vi "Transcriptor LabVIEW to VHDL code Step 1 and 2 Wires Declarations and Assignements.vi"(8 "error in":errorcluster, 11 "Diagram in":refnum<vi>) -> (1 "wires with enabled breakpoints":string[](array[string]), 2 "wires declarations":string[](array[string]), 3 "end loop refs.":string[](array[string]))   [LabVIEW 2018]
uses:
  <vilib>/Utility/miscctls.llb/LVBreakpointStatusEnum.ctl
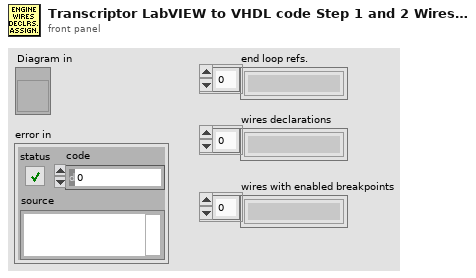
[diagram p1: front panel]
types:
  T1 = typedef "LVBreakpointStatusEnum.ctl" = enum8{"Cleared Break", "Enabled Break", "Disabled Break"}
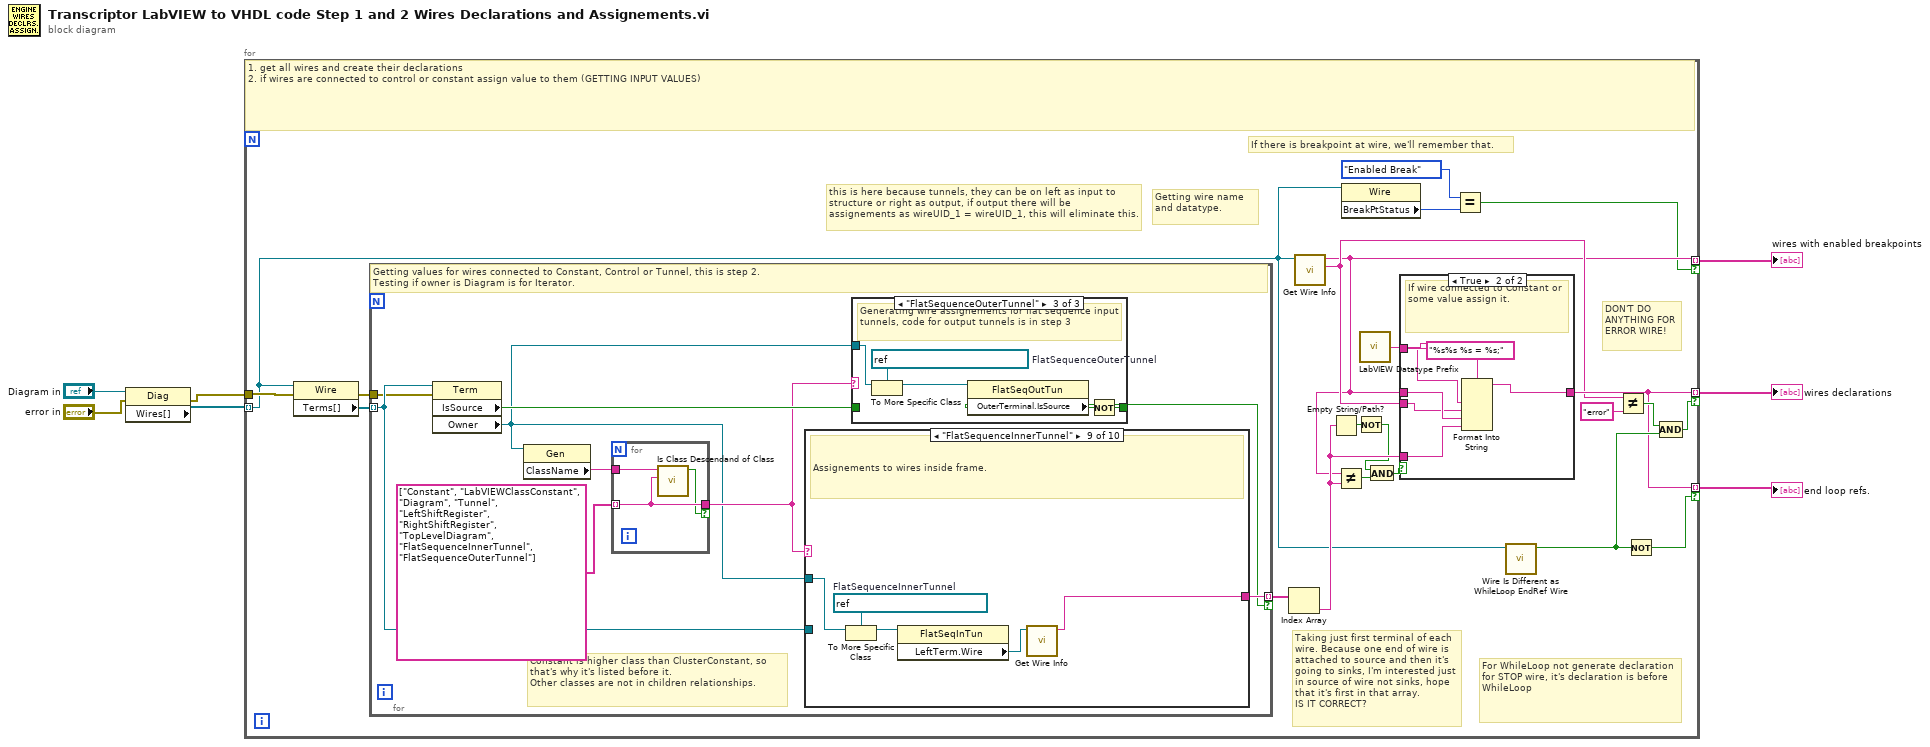
[diagram p0: block diagram]
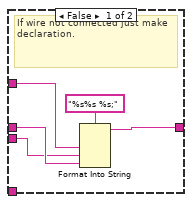
[diagram p2: hidden frame]
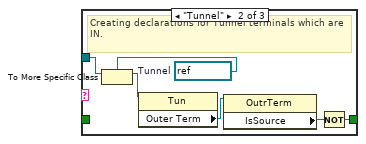
[diagram p4: hidden frame]
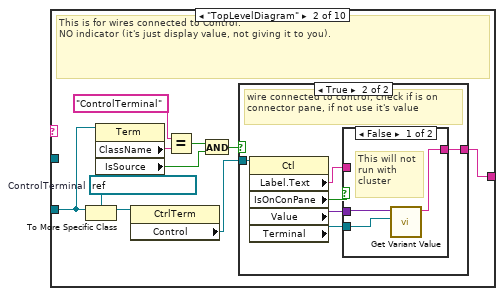
[diagram p6: hidden frame]
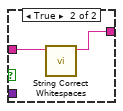
[diagram p8: hidden frame]
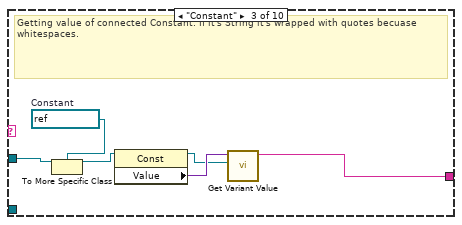
[diagram p9: hidden frame]
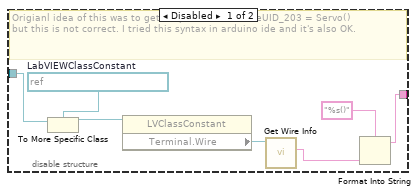
[diagram p11: hidden frame]
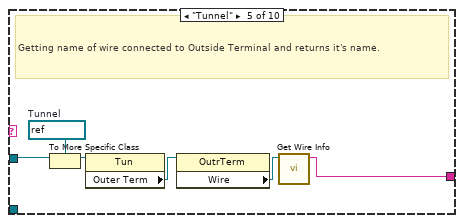
[diagram p12: hidden frame]
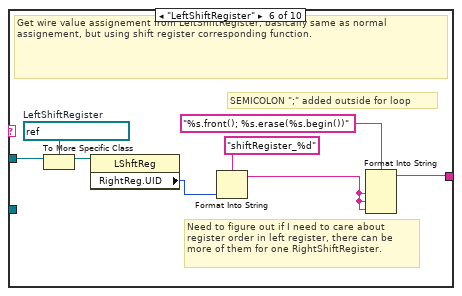
[diagram p13: hidden frame]
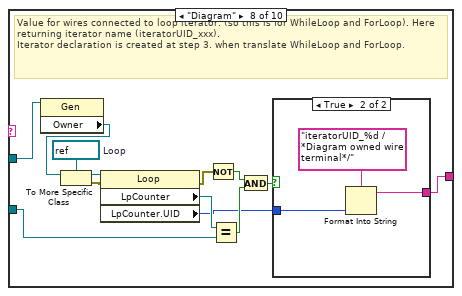
[diagram p15: hidden frame]
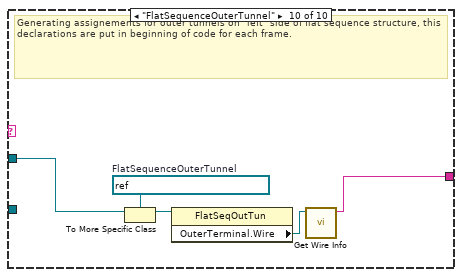
[diagram p17: hidden frame]
diagram:
  n1 = property class="Diag"(reference="Diagram in", error in="error in") -> (error out=w3:errorcluster, "Wires[]"=w2:refnum<vi>[])  [unwired: 1 out]
  n2 = for {
    tunnel: w2 -> [w12] mode=indexing
    tunnel: [w19] -> w7 mode=indexing if=w21
    tunnel: w3 -> [w25]
    tunnel: [w19] -> w6 mode=indexing if=w18
    tunnel: [w9] -> w1 mode=indexing if=w8
    # "If there is breakpoint at wire, we'll remember that."
    # "this is here because tunnels, they can be on left as input to structure or right as output, if output there will be assignements as wireUID_1 = wireUID_1, this will eliminate this."
    # "Getting wire name and datatype."
    # "For WhileLoop not generate declaration for STOP wire, it's declaration is before WhileLoop"
    # "Taking just first terminal of each wire. Because one end of wire is attached to source and then it's going to sinks, I'm interested just in source of wire not sinks, hope that it's first in that array.\nIS IT CORRECT?"
    # "DON'T DO ANYTHING FOR ERROR WIRE!"
    # "1. get all wires and create their declarations\n2. if wires are connected to control or constant assign value to them (GETTING INPUT VALUES)"
    n3 = property class="Wire"(reference=w12, error in=w25) -> (error out=w24:errorcluster, "Terms[]"=w29:refnum<vi>[])  [unwired: 1 out]
    n4 = for {
      tunnel: w29 -> [w48] mode=indexing
      tunnel: [w49] -> w28 mode=indexing if=w46
      tunnel: w24 -> [w47]
      # "Constant is higher class than ClusterConstant, so that's why it's listed before it.\nOther classes are not in children relationships."
      # "Getting values for wires connected to Constant, Control or Tunnel, this is step 2.\nTesting if owner is Diagram is for Iterator."
      n5 = property class="Term"(reference=w48, error in=w47) -> ("IsSource"=w45:bool, "Owner"=w41:refnum<vi>)  [unwired: 2 out]
      n6 = property class="Gen"(reference=w41) -> ("ClassName"=w43:string)  [unwired: 1 in, 2 out]
      n7 = for {
        tunnel: string[] ["Constant", "LabVIEWClassConstant", "Diagram", "Tunnel", "LeftShiftRegister", "RightShiftRegister", "TopLevelDiagram", "FlatSequenceInnerTunnel", "FlatSequenceOuterTunnel"] -> [w51] mode=indexing
        tunnel: w43 -> [w52]
        tunnel: [w51] -> w42 if=w50
        n8 = call "Is Class Descendand of Class.vi"("Parent ClassName"=w51, "ClassName"=w52) -> ("is Class descendant?"=w50:bool)  [unwired: 8 in, 1 out]
      }
      n9 = case shown="\"FlatSequenceInnerTunnel\"" w42 {
        tunnel: w41 -> [_ _ w91 w93 w105 w112 _ w127 w131 w136]
        tunnel: [_ w72 w88 w92 w101 w107 _ w117 w132 w138] -> w49
        tunnel: w48 -> [_ w70 _ _ _ _ _ w123 _ _]
        frame Default {
          # "If wire is not wired to anything from what I have to read value, output is default Variant value (hope that is empty Variant), and there will be just wire declaration without assignement in generated code."
        }
        frame "TopLevelDiagram" {
          w74 = refnum<vi> refnum  # ControlTerminal
          # "This is for wires connected to Control.\nNO indicator (it's just display value, not giving it to you)."
          n10 = To More Specific Class(target class=w74, reference=w70) -> (specific class reference=w73:refnum<vi>)  [unwired: 1 in, 1 out]
          n11 = property class="Term"(reference=w70) -> ("ClassName"=w69:string, "IsSource"=w65:bool)  [unwired: 1 in, 2 out]
          n12 = property class="CtrlTerm"(reference=w73) -> ("Control"=w68:refnum<vi>)  [unwired: 1 in, 2 out]
          n13 = Equal?(x="ControlTerminal", y=w69) -> (x = y?=w66:bool)
          n14 = And(x=w66, y=w65) -> (x .and. y?=w67:bool)
          n15 = case shown="True" w67 {
            tunnel: [_ w78] -> w72
            tunnel: w68 -> [_ w80]
            frame False {
              # "wire connected to indicator, do nothing"
            }
            frame True {
              # "wire connected to control, check if is on connector pane, if not use it's value"
              n16 = property class="Ctl"(reference=w80) -> ("Label.Text"=w79:string, "IsOnConPane"=w77:bool, "Value"=w76:variant, "Terminal"=w75:refnum<vi>)  [unwired: 1 in, 2 out]
              n17 = case shown="False" w77 {
                tunnel: w79 -> [_ w85]
                tunnel: [w82 w84] -> w78
                tunnel: w76 -> [w83 _]
                tunnel: w75 -> [w81 _]
                frame False {
                  # "This will not\nrun with\ncluster"
                  n18 = call "Get Variant Value.vi"("GObj Refnum"=w81, "Variant in"=w83) -> ("Variant value as string"=w82:string)  [unwired: 9 in]
                }
                frame True {
                  n19 = call "String Correct Whitespaces.vi"("String in"=w85) -> ("String out"=w84:string)  [unwired: 10 in]
                }
              }
            }
          }
        }
        frame "Constant" {
          w90 = refnum<vi> refnum  # Constant
          # "Getting value of connected Constant. If it's String it's wrapped with quotes becuase whitespaces."
          n20 = To More Specific Class(target class=w90, reference=w91) -> (specific class reference=w89:refnum<vi>)  [unwired: 1 in, 1 out]
          n21 = property class="Const"(reference=w89) -> (reference out=w86:refnum<vi>, "Value"=w87:variant)  [unwired: 1 in, 1 out]
          n22 = call "Get Variant Value.vi"("GObj Refnum"=w86, "Variant in"=w87) -> ("Variant value as string"=w88:string)  [unwired: 9 in]
        }
        frame "LabVIEWClassConstant" {
          # "For class constant connected to wire there is nothing to get, we have to in the end obtain just normal C++ object declaration ie. for Servo class:\nServo wireUID_203;"
          n23 = disable-structure shown="Enabled" {
            disable-tunnel: w93 -> [w100 _]
            disable-tunnel: [w95 _] -> w92
            frame Disabled {
              w99 = refnum<vi> refnum  # LabVIEWClassConstant
              # "Origianl idea of this was to get output as Servo wireUID_203 = Servo()\nbut this is not correct. I tried this syntax in arduino ide and it's also OK."
              n24 = To More Specific Class(target class=w99, reference=w100) -> (specific class reference=w98:refnum<vi>)  [unwired: 1 in, 1 out]
              n25 = property class="LVClassConstant"(reference=w98) -> ("Terminal.Wire"=w97:refnum<vi>)  [unwired: 1 in, 2 out]
              n26 = call "Get Wire Info.vi"("Wire"=w97) -> ("wire datatype"=w94:string)  [unwired: 9 in, 1 out]
              n27 = Format Into String(format string="%s()", w94) -> (resulting string=w95:string)  [unwired: 2 in, 1 out]
            }
            frame Enabled {
              # "Nothing to return, so in the end object wire declaration is without initilization (we are working normal memory of MCU NOT in stack!)"
            }
          }
        }
        frame "Tunnel" {
          w106 = refnum<vi> refnum  # Tunnel
          # "Getting name of wire connected to Outside Terminal and returns it's name."
          n28 = To More Specific Class(target class=w106, reference=w105) -> (specific class reference=w104:refnum<vi>)  [unwired: 1 in, 1 out]
          n29 = property class="Tun"(reference=w104) -> ("Outer Term"=w103:refnum<vi>)  [unwired: 1 in, 2 out]
          n30 = property class="OutrTerm"(reference=w103) -> ("Wire"=w102:refnum<vi>)  [unwired: 1 in, 2 out]
          n31 = call "Get Wire Info.vi"("Wire"=w102) -> ("wire label"=w101:string)  [unwired: 9 in, 1 out]
        }
        frame "LeftShiftRegister" {
          w114 = refnum<vi> refnum  # LeftShiftRegister
          # "SEMICOLON \";\" added outside for loop"
          # "Need to figure out if I need to care about register order in left register, there can be more of them for one RightShiftRegister."
          # "Get wire value assignement from LeftShiftRegister, basically same as normal assignement, but using shift register corresponding function."
          n32 = To More Specific Class(target class=w114, reference=w112) -> (specific class reference=w113:refnum<vi>)  [unwired: 1 in, 1 out]
          n33 = property class="LShftReg"(reference=w113) -> ("RightReg.UID"=w110:i32)  [unwired: 1 in, 2 out]
          n34 = Format Into String(format string="shiftRegister_%d", w110) -> (resulting string=w108:string)  [unwired: 2 in, 1 out]
          n35 = Format Into String(format string="%s.front(); %s.erase(%s.begin())", w108, w108, w108) -> (resulting string=w107:string)  [unwired: 2 in, 1 out]
        }
        frame "RightShiftRegister" {
          # "For RightShiftRegister there is nothing to do, no init value, so this left blank."
        }
        frame "Diagram" {
          w126 = refnum<vi> refnum  # Loop
          # "Value for wires connected to loop iterator. (so this is for WhileLoop and ForLoop). Here returning iterator name (iteratorUID_xxx).\nIterator declaration is created at step 3. when translate WhileLoop and ForLoop."
          n36 = property class="Gen"(reference=w127) -> ("Owner"=w115:refnum<vi>)  [unwired: 1 in, 2 out]
          n37 = To More Specific Class(target class=w126, reference=w115) -> (specific class reference=w125:refnum<vi>, error out=w122:errorcluster)  [unwired: 1 in]
          n38 = property class="Loop"(reference=w125, error in=w122) -> (error out=w121:errorcluster, "LpCounter"=w124:refnum<vi>, "LpCounter.UID"=w116:i32)  [unwired: 1 out]
          n39 = Not(x=w121) -> (.not. x?=w120:bool)
          n40 = Equal?(x=w124, y=w123) -> (x = y?=w119:bool)
          n41 = And(x=w120, y=w119) -> (x .and. y?=w118:bool)
          n42 = case shown="True" w118 {
            tunnel: [_ w130] -> w117
            tunnel: w116 -> [_ w128]
            frame False {
            }
            frame True {
              n43 = Format Into String(format string="iteratorUID_%d /*Diagram owned wire terminal*/", w128) -> (resulting string=w130:string)  [unwired: 2 in, 1 out]
            }
          }
        }
        frame "FlatSequenceInnerTunnel" {
          w135 = refnum<vi> refnum  # FlatSequenceInnerTunnel
          # "Assignements to wires inside frame."
          n44 = To More Specific Class(target class=w135, reference=w131) -> (specific class reference=w134:refnum<vi>)  [unwired: 1 in, 1 out]
          n45 = property class="FlatSeqInTun"(reference=w134) -> ("LeftTerm.Wire"=w133:refnum<vi>)  [unwired: 1 in, 2 out]
          n46 = call "Get Wire Info.vi"("Wire"=w133) -> ("wire label"=w132:string)  [unwired: 9 in, 1 out]
        }
        frame "FlatSequenceOuterTunnel" {
          w140 = refnum<vi> refnum  # FlatSequenceOuterTunnel
          # "Generating assignements for outer tunnels on \"left\" side of flat sequence structure, this declarations are put in beginning of code for each frame."
          n47 = To More Specific Class(target class=w140, reference=w136) -> (specific class reference=w139:refnum<vi>)  [unwired: 1 in, 1 out]
          n48 = property class="FlatSeqOutTun"(reference=w139) -> ("OuterTerminal.Wire"=w137:refnum<vi>)  [unwired: 1 in, 2 out]
          n49 = call "Get Wire Info.vi"("Wire"=w137) -> ("wire label"=w138:string)  [unwired: 9 in, 1 out]
        }
      }
      n50 = case shown="\"FlatSequenceOuterTunnel\"" w42 {
        tunnel: [w53 w54 w61] -> w46
        tunnel: w45 -> [w53 _ _]
        tunnel: w41 -> [_ w56 w62]
        frame Default {
          # "For all others Terminal.Owner don't need to do anything else."
        }
        frame "Tunnel" {
          w58 = refnum<vi> refnum  # Tunnel
          # "Creating declarations for Tunnel terminals which are IN."
          n51 = To More Specific Class(target class=w58, reference=w56) -> (specific class reference=w59:refnum<vi>)  [unwired: 1 in, 1 out]
          n52 = property class="Tun"(reference=w59) -> ("Outer Term"=w57:refnum<vi>)  [unwired: 1 in, 2 out]
          n53 = property class="OutrTerm"(reference=w57) -> ("IsSource"=w55:bool)  [unwired: 1 in, 2 out]
          n54 = Not(x=w55) -> (.not. x?=w54:bool)
        }
        frame "FlatSequenceOuterTunnel" {
          w63 = refnum<vi> refnum  # FlatSequenceOuterTunnel
          # "Generating wire assignements for flat sequence input tunnels, code for output tunnels is in step 3"
          n55 = To More Specific Class(target class=w63, reference=w62) -> (specific class reference=w64:refnum<vi>)  [unwired: 1 in, 1 out]
          n56 = property class="FlatSeqOutTun"(reference=w64) -> ("OuterTerminal.IsSource"=w60:bool)  [unwired: 1 in, 2 out]
          n57 = Not(x=w60) -> (.not. x?=w61:bool)
        }
      }
    }
    n58 = Index Array(array=w28) -> (element=w17:string)  [unwired: 1 in]
    n59 = call "Get Wire Info.vi"("Wire"=w12) -> ("wire datatype"=w16:string, "wire label"=w9:string)  [unwired: 9 in]
    n60 = Empty String/Path?(string/path=w17) -> (empty?=w27:bool)
    n61 = Not Equal?(x=w9, y=w17) -> (x != y?=w15:bool)
    n62 = property class="Wire"(reference=w12) -> ("BreakPtStatus"=w11:T1)  [unwired: 1 in, 2 out]
    n63 = Not(x=w27) -> (.not. x?=w14:bool)
    n64 = call "LabVIEW Datatype Prefix.vi"() -> ("datatype prefix"=w23:string)
    n65 = And(x=w14, y=w15) -> (x .and. y?=w13:bool)
    n66 = case shown="True" w13 {
      tunnel: w9 -> [w32 w37]
      tunnel: w16 -> [w31 w36]
      tunnel: w17 -> [_ w39]
      tunnel: [w33 w38] -> w19
      tunnel: w23 -> [w30 w35]
      frame False {
        # "If wire not connected just make declaration."
        n67 = Format Into String(format string="%s%s %s;", w30, w31, w32) -> (resulting string=w33:string)  [unwired: 2 in, 1 out]
      }
      frame True {
        # "If wire connected to Constant or some value assign it."
        n68 = Format Into String(format string="%s%s %s = %s;", w35, w36, w37, w39) -> (resulting string=w38:string)  [unwired: 2 in, 1 out]
      }
    }
    n69 = Equal?(x=LVBreakpointStatusEnum."Enabled Break", y=w11) -> (x = y?=w8:bool)
    n70 = call "Wire Is Different as WhileLoop EndRef Wire.vi"("Wire in"=w12) -> ("is different than WhileLoop endref?"=w20:bool)  [unwired: 10 in]
    n71 = Not Equal?(x=w16, y="error") -> (x != y?=w22:bool)
    n72 = Not(x=w20) -> (.not. x?=w18:bool)
    n73 = Compound Arithmetic op=AND(w22, w20) -> (w21:bool)
  }
  "wires declarations" <- w7
  "end loop refs." <- w6
  "wires with enabled breakpoints" <- w1
